vi "crio_RT_LAC_closed_loop.vi"() -> ()   [LabVIEW 2019]
uses:
  <vilib>/Platform/TimedLoop/XDataNode/timing_clust.ctl
  <vilib>/Platform/TimedLoop/XDataNode/nitl_modes.ctl
  <vilib>/Platform/TimedLoop/XDataNode/wakeup.ctl
  <vilib>/FPGAPlugInAG/cRIO-9074/niLvFpga_Open_cRIO-9074.vi
  <vilib>/rvi/interface/common/dynamic/niFpgaDynamicAddResources.vi
  <vilib>/Utility/error.llb/Error Cluster From Error Code.vi
  <vilib>/rvi/errors/niLvFpgaAdjustHostInterfaceError.vi
  <vilib>/FPGAPlugInAG/Dynamic/niLvFpga_Close_Dynamic.vi
  <vilib>/rvi/interface/nirviOpenFPGA/nirviOpenFPGA.xnode
  FPGA Bitfiles/gpass2_FPGATarget2_crioFPGALACPWMef_GNxQiAuroRM.lvbitx
  crio_FPGA_LAC_PWM_efficient.vi
  <vilib>/rvi/interface/nirviReadWriteControl/nirviReadWriteControl.xnode
  <vilib>/platform/TimedLoop/XDataNode/XDataNode.xnode
  <vilib>/rvi/interface/nirviCloseFPGA/nirviCloseFPGA.xnode
  NiFpgaLv.dll
  <vilib>/rvi/interface/Simulation/niFpgaSimulationCallBeginRW.vi
  <vilib>/Platform/TimedLoop/XDataNode/XDNodeRunTimeDep.lvlib
panel:
  in  "output range":T1={"output high (Inf)"=0.5, "output low (-Inf)"=-0.5}
  in  "Autolock":bool
  in  "stop":bool=TRUE
  out "Measured Velocity (Counts/Interval)":i32
  out "Controller PWM Output":sgl=-0.5
  out "Measured Position":i32=3
  in  "Loop Period":i64=1000
  out "velocity":i32(graph)
  out "controller pwm output":sgl(graph)=-0.5
  out "measured position":i32(graph)=3
  in  "manual control":T2 {"manual input (0)" scale=-1.0..1.0}
  in  "Position Reset":bool
  in  "Gains":T3={"proportional gain"=0.97979796, "integral gain"=0.530303} {"proportional gain" scale=0.0..1.0; "integral gain" scale=0.0..1.0}
  in  "Velocity Interval (uSec)":u32=1000
  in  "setpoint":i32(slide) scale=0.0..4500.0
  out "Actual Gain":T3={"proportional gain"=0.0009797979, "integral gain"=5.30303e-09}
  in  "Gain Scaler":T3={"proportional gain"=1000.0, "integral gain"=100000000.0}
  in  "PWM Frequency (default 2kHz) for LAC":i32=2000
  # "full extension is about 4961"
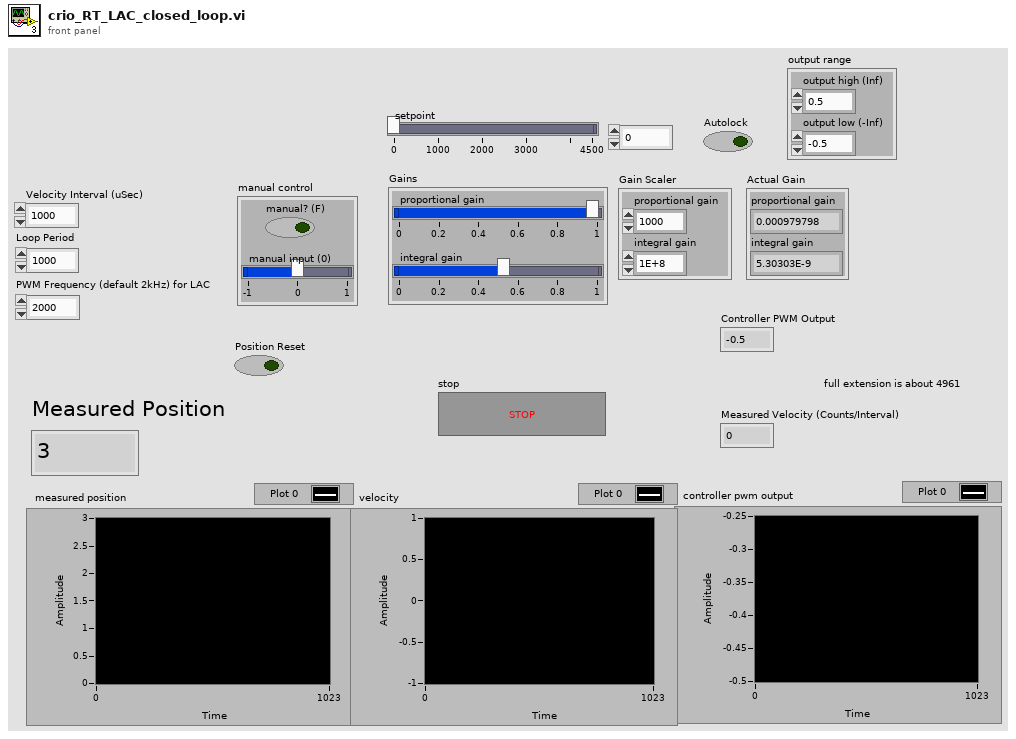
[diagram p1: front panel]
types:
  T1 = cluster{"output high (Inf)":sgl, "output low (-Inf)":sgl}
  T2 = cluster{"manual? (F)":bool, "manual input (0)":sgl}
  T3 = cluster{"proportional gain":sgl, "integral gain":sgl}
  T4 = typedef "XDNodeRunTimeDep.lvlib/timing_clust.ctl" = cluster{"Expected End [f-1]":u64, "Actual End [f-1]":u64, "Finished Late? [f-1]":bool, "Expected End [i-1]":u64, "Actual End [i-1]":u64, "Finished Late? [i-1]":bool, "Expected Start [i]":u64, "Actual Start [i]":u64, "Expected Start [f]":u64, "Actual Start [f]":u64, "Source Name":string, "Structure Name":string, "Period":i64, "Deadline":i64, "Offset":i64, "Start":i64, "Priority":i32, "Timeout":i32, "Mode":T5, "Wakeup Reason":T6, "Error":errorcluster, "Source Type":string, "Secondary Source Type":string, "Global End Time":u64, "Global Start Time":u64, "Frame Duration":u64, "Iteration Duration":u64, "Assigned CPU":i32, "I/O Scan Engine Mode":u32}
  T5 = typedef "XDNodeRunTimeDep.lvlib/nitl_modes.ctl" = enum32{"No Change", "Process missed periods, maintain original phase", "Discard missed periods, maintain original phase", "Process missed periods, ignore original phase", "Discard missed periods, ignore original phase"}
  T6 = typedef "XDNodeRunTimeDep.lvlib/wakeup.ctl" = enum32{"Normal", "Aborted", "Asynchronous wakeup", "Timing source error", "Timed loop error", "Timeout"}
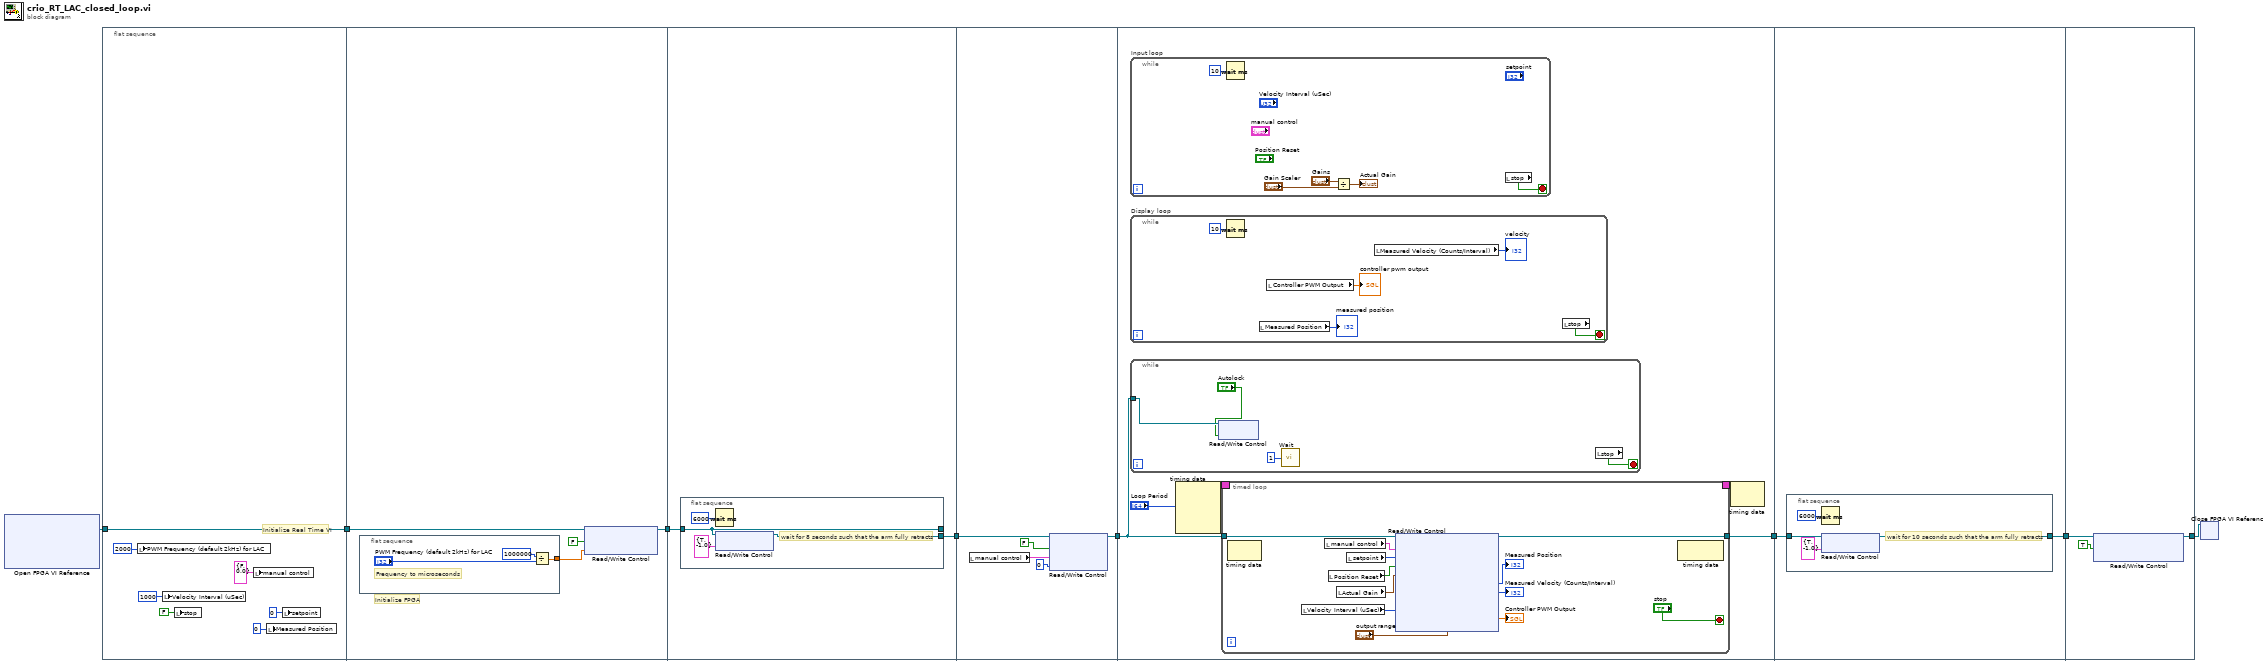
[diagram p0: block diagram]
diagram:
  n1 = xnode "Open FPGA VI Reference"() -> ("FPGA VI Reference Out"=w6:refnum<k20>)  [unwired: 2 in, 1 out]
  n2 = flat-sequence {
    tunnel: [w14] -> w8
    tunnel: w6 -> [w14]
    tunnel: w8 -> [w18]
    tunnel: [w17] -> w2
    tunnel: w2 -> [w24]
    tunnel: [w23] -> w1
    tunnel: [w33] -> w7
    tunnel: w1 -> [w29]
    tunnel: w7 -> [w34]
    tunnel: [w35] -> w4
    tunnel: w4 -> [w71]
    tunnel: [w72] -> w3
    tunnel: w3 -> [w79]
    tunnel: [w77] -> w5
    frame #0 {
      # "Initialize Real Time VI"
      n3 = local write "PWM Frequency (default 2kHz) for LAC"(2000 ("PWM Frequency")) -> ()
      n4 = local write "Velocity Interval (uSec)"(u32 1000 ("Velocity Interval (uSec)")) -> ()
      n5 = local write "stop"(FALSE ("stop")) -> ()
      n6 = local write "manual control"(T2 {"manual? (F)"=FALSE, "manual input (0)"=0.0} ("manual control")) -> ()
      n7 = local write "Measured Position"(0 ("Measured Position")) -> ()
      n8 = local write "setpoint"(0 ("setpoint")) -> ()
    }
    frame #1 {
      # "Initialize FPGA"
      n9 = flat-sequence {
        tunnel: [w20] -> w16
        frame #0 {
          # "Frequency to microseconds"
          n10 = Divide(x=1000000, y="PWM Frequency (default 2kHz) for LAC") -> (x/y=w20:dbl)
        }
      }
      n11 = xnode "Read/Write Control"("FPGA VI Reference In"=w18, "stop"=FALSE, "DC PWM Period (us)"=w16) -> ("FPGA VI Reference Out"=w17:refnum<k20>)  [unwired: 1 in, 1 out]
    }
    frame #2 {
      n12 = flat-sequence {
        tunnel: [w26] -> _
        tunnel: w24 -> [w26]
        tunnel: [w25] -> w23
        frame #0 {
          # "wait for 8 seconds such that the arm fully retracts"
          n13 = Wait (ms)(milliseconds to wait=u32 6000) -> ()  [unwired: 1 out]
          n14 = xnode "Read/Write Control"("FPGA VI Reference In"=w26, "manual control"=T2 {"manual? (F)"=TRUE, "manual input (0)"=-1.0}) -> ("FPGA VI Reference Out"=w25:refnum<k20>)  [unwired: 1 in, 1 out]
        }
      }
    }
    frame #3 {
      n15 = local read "manual control"() -> (w30:T2)
      n16 = xnode "Read/Write Control"("FPGA VI Reference In"=w29, "Position Reset"=FALSE, "manual control"=w30, "setpoint"=0) -> ("FPGA VI Reference Out"=w33:refnum<k20>)  [unwired: 1 in, 1 out]
    }
    frame #4 {
      n17 = while "Input loop" {
        stop <- w46 stop-if-true
        n18 = Wait (ms)(milliseconds to wait=u32 10) -> ()  [unwired: 1 out]
        n19 = Divide(x="Gains", y="Gain Scaler") -> (x/y=→"Actual Gain":T3)
        n20 = local read "stop"() -> (w46:bool)
      }
      n21 = while "Display loop" {
        stop <- w51 stop-if-true
        n22 = Wait (ms)(milliseconds to wait=u32 10) -> ()  [unwired: 1 out]
        n23 = local read "Measured Position"() -> (→"measured position":i32)
        n24 = local read "Controller PWM Output"() -> (→"controller pwm output":sgl)
        n25 = local read "Measured Velocity (Counts/Interval)"() -> (→"velocity":i32)
        n26 = local read "stop"() -> (w51:bool)
      }
      n27 = while {
        tunnel: w34 -> [w40]
        stop <- w42 stop-if-true
        n28 = xnode "Read/Write Control"("FPGA VI Reference In"=w40, "LAC Lock"="Autolock") -> ()  [unwired: 1 in, 2 out]
        n29 = call "Wait"("Count(mSec)"=u32 1) -> ()  [unwired: 1 out]
        n30 = local read "stop"() -> (w42:bool)
      }
      n31 = node-c288("Loop Period") -> (w38:T4)  [unwired: 3 in]
      n32 = timed-loop {
        timing: w38 -> [_]
        timing-out: [_] -> w37
        tunnel: w34 -> [w63]
        tunnel: [w54] -> w35
        stop <- "stop" stop-if-true
        n33 = node-c288() -> ()  [unwired: 1 in, 1 out]
        n34 = local read "Velocity Interval (uSec)"() -> (w55:u32)
        n35 = local read "manual control"() -> (w56:T2)
        n36 = local read "Position Reset"() -> (w59:bool)
        n37 = local read "Actual Gain"() -> (w58:T3)
        n38 = local read "setpoint"() -> (w57:i32)
        n39 = xnode "Read/Write Control"("FPGA VI Reference In"=w63, "manual control"=w56, "setpoint"=w57, "Position Reset"=w59, "gains"=w58, "Velocity Interval (uSec)"=w55, "output range"="output range") -> ("FPGA VI Reference Out"=w54:refnum<k20>, "Position (Counts)"=→"Measured Position":i32, "Velocity (Counts/Interval)"=→"Measured Velocity (Counts/Interval)":i32, "ControllerPWM Output"=→"Controller PWM Output":sgl)  [unwired: 1 in, 2 out]
        n40 = node-c288() -> ()  [unwired: 1 in, 1 out]
      }
      n41 = node-c288(w37) -> ()  [unwired: 1 out]
    }
    frame #5 {
      n42 = flat-sequence {
        tunnel: [w76] -> w72
        tunnel: w71 -> [w75]
        frame #0 {
          # "wait for 10 seconds such that the arm fully retracts"
          n43 = xnode "Read/Write Control"("FPGA VI Reference In"=w75, "manual control"=T2 {"manual? (F)"=TRUE, "manual input (0)"=-1.0}) -> ("FPGA VI Reference Out"=w76:refnum<k20>)  [unwired: 1 in, 1 out]
          n44 = Wait (ms)(milliseconds to wait=u32 6000) -> ()  [unwired: 1 out]
        }
      }
    }
    frame #6 {
      n45 = xnode "Read/Write Control"("FPGA VI Reference In"=w79, "stop"=TRUE) -> ("FPGA VI Reference Out"=w77:refnum<k20>)  [unwired: 1 in, 2 out]
    }
  }
  n46 = xnode "Close FPGA VI Reference"("FPGA VI Reference In"=w5) -> ()  [unwired: 1 in, 1 out]
